vi "zmq_bind_random.vi"(4 "error in":errorcluster, 5 "base":string="tcp://*", 7 "socket in":refnum<class "Socket.lvclass">) -> (0 "error out":errorcluster, 1 "endpoint":string, 2 "port":u16, 3 "socket out":refnum<class "Socket.lvclass">)   [LabVIEW 2025, in "ZeroMQ.lvlib" / "Socket.lvclass"]
doc: "Binds a socket to an unused ephemeral port, returning the port number. The port number is obtained from the OS by LabVIEW (see the documentation for UDP Open).\n\nSee also the documentation for zmq_bind"
uses:
  Socket.lvclass
  Socket.lvclass/Socket.ctl
panel:
  # "ØMQ"
  # "labview"
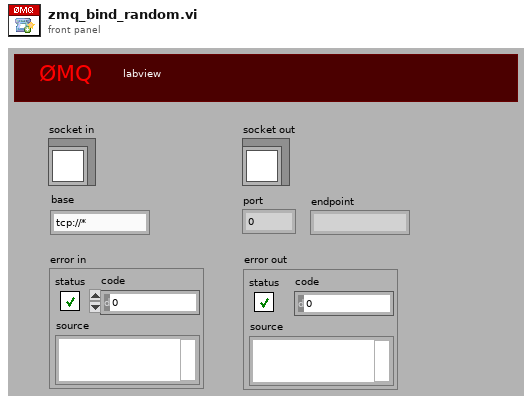
[diagram p1: front panel]
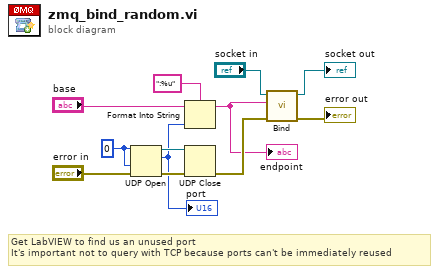
[diagram p0: block diagram]
diagram:
  w5 = u16 0 ("port")
  # "Get LabVIEW to find us an unused port\nIt's important not to query with TCP because ports can't be immediately reused"
  n1 = UDP Open(8:"error in", 9:w5, 11:w5) -> (port=w11:refnum<k16>, 0:w12:errorcluster, 2:w10:u16)  [unwired: 2 in]
  "port" <- w10
  n2 = Format Into String(format string=":%u", initial string="base", w10) -> (resulting string=w7:string)  [unwired: 1 in, 1 out]
  "endpoint" <- w7
  n3 = UDP Close(connection ID=w11, 8:w12) -> (error out=w8:errorcluster)  [unwired: 1 out]
  n4 = call "Bind.vi"("error in"=w8, "endpoint"=w7, "socket in"="socket in") -> ("error out"=→"error out":errorcluster, "socket out"=→"socket out":refnum<class "Socket.lvclass">)  [unwired: 7 in]
